vi "Target Main.vi"() -> ()   [LabVIEW 2013]
doc: "This application launches and executes the Tag Bus Data framework configuration for the specified target alias. This is a simple example of the framework API functions, but may also be a suitable starting point for a Host UI or Thick Client that is running a local version of the framework."
uses:
  <vilib>/NI/Module Execution Interface/Engine Runtime/Execution States.ctl
  <vilib>/NI/Module Execution Interface/Engine Runtime/Fault.ctl
  <vilib>/NI/Tag Bus Module Framework/runtime/error classification.ctl
  <vilib>/NI/Module Execution Interface/Engine Runtime/Engine Runtime Interface.lvclass
  <vilib>/userdefined/High Color/nirio_resource_hc.ctl
  <vilib>/NI/DCAF/Tag Editor Core/Framework Configuration Classes/target runtime/PL_Target Runtime.lvclass
  <vilib>/NI/Tag Bus Module Framework/FPGA manager/FPGA manager.lvlib
  <vilib>/rvi/interface/nirviOpenFPGA/nirviOpenFPGA.xnode
  <vilib>/NI/Tag Bus Module Framework/FPGA manager/methods.ctl
  <vilib>/NI_Real-Time Target Support.lvlib
  <vilib>/NI/Tag Bus Module Framework/runtime/TBM module execution interface.lvclass
panel:
  in  "configuration file path":path=path "/home/lvuser/DCAFshm.pcfg"
  in  "target alias":string="cRIO"
  out "engine status":T4(array[cluster])
  out "stop":bool
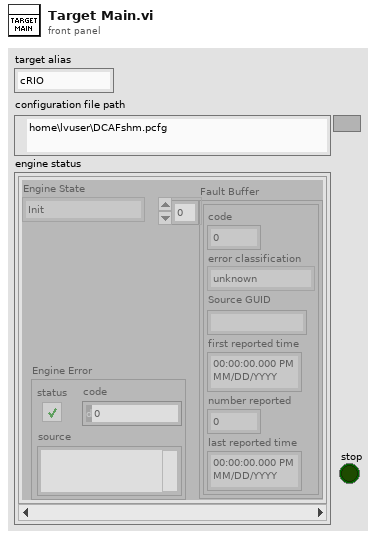
[diagram p1: front panel]
types:
  T1 = typedef "Engine Runtime Interface.lvclass/Execution States.ctl" = enum16{"Init", "Pre-Operational", "Safe-Operational", "Operational", "Stopped"}
  T2 = typedef "Engine Runtime Interface.lvclass/Fault.ctl" = cluster{"code":i32, "error classification":T3, "Source GUID":string, "first reported time":timestamp, "number reported":u32, "last reported time":timestamp}
  T3 = typedef "TBM module execution interface.lvclass/error classification.ctl" = enum16{"unknown", "none", "trivial", "recoverable", "critical"}
  T4 = cluster{"Engine State":T1, "Fault Buffer":T2[], "Engine Error":errorcluster}[]
  T5 = typedef "FPGA manager.lvlib/methods.ctl" = enum16{"initialize bitfile", "cache bitfile", "locate bitfile", "close bitfile", "clear manager"}
  T6 = typedef "nirio_resource_hc.ctl" = tag
  T7 = cluster{"Engine State":T1, "faults":T2[], "Engine Error":errorcluster}
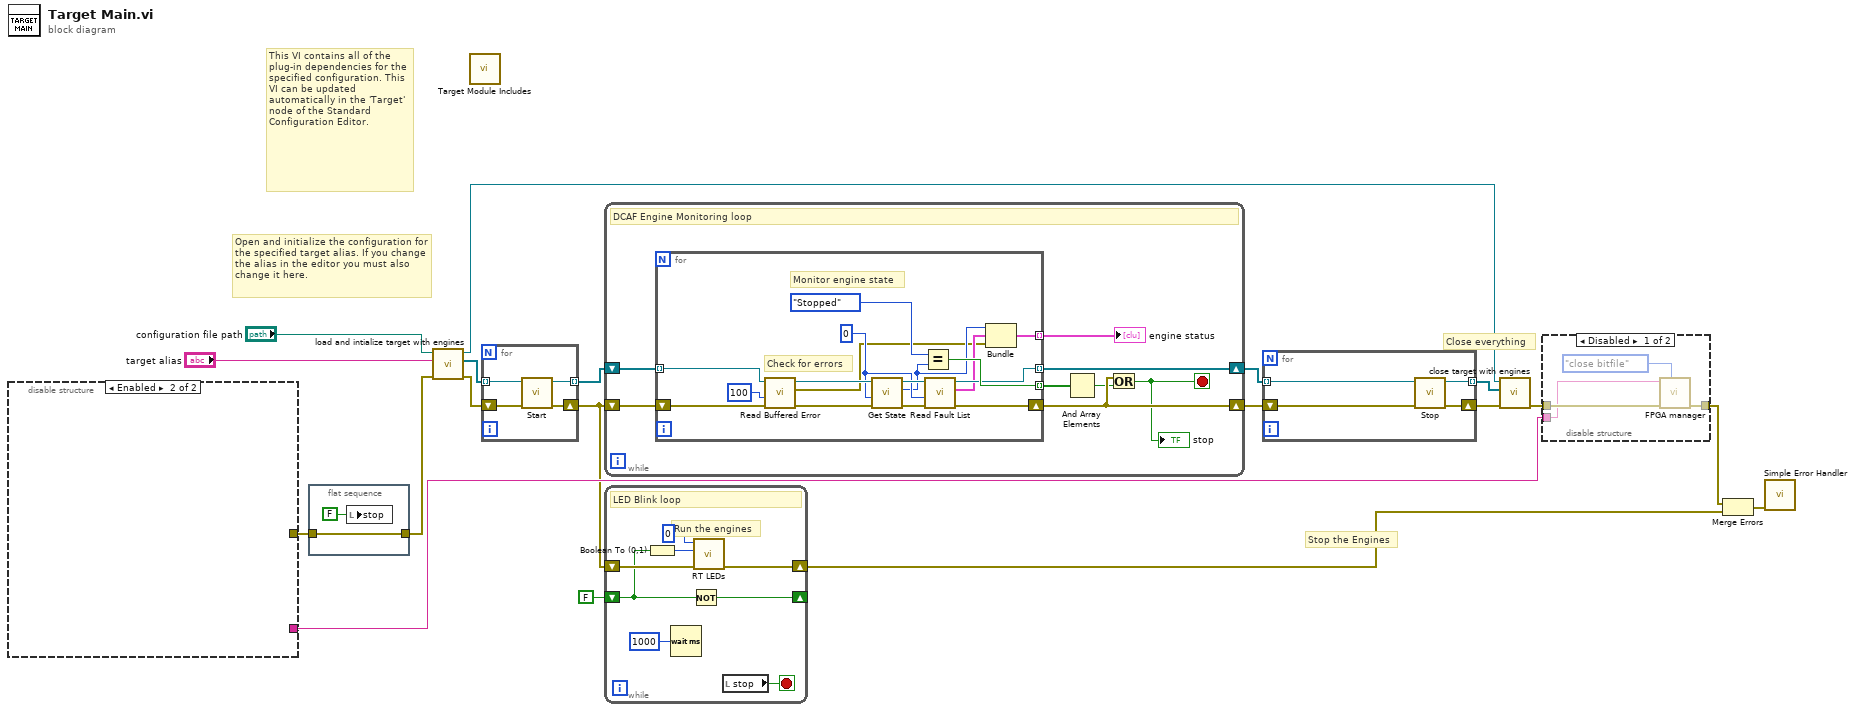
[diagram p0: block diagram]
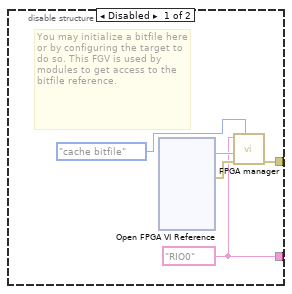
[diagram p3: hidden frame]
diagram:
  # "Open and initialize the configuration for the specified target alias. If you change the alias in the editor you must also change it here."
  # "Close everything"
  # "Stop the Engines"
  # "This VI contains all of the plug-in dependencies for the specified configuration. This VI can be updated automatically in the 'Target' node of the Standard Configuration Editor."
  # "Run the engines"
  n1 = disable-structure shown="Enabled" {
    disable-tunnel: [w24 _] -> w3
    disable-tunnel: [w20 _] -> w9
    frame Disabled {
      w20 = T6 "RIO0" ("RIO resource")
      # "You may initialize a bitfile here or by configuring the target to do so. This FGV is used by modules to get access to the bitfile reference."
      n2 = xnode "Open FPGA VI Reference"() -> ("FPGA VI Reference Out"=w22:refnum<k20>, "error out"=w23:errorcluster)  [unwired: 2 in]
      n3 = call <vilib>:"FPGA manager.vi"("action"=methods."cache bitfile", "error in"=w23, "bitfile to cache"=w22, "RIO resource"=w20) -> ("error out"=w24:errorcluster)  [unwired: 5 in, 2 out]
    }
    frame Enabled {
    }
  }
  n4 = flat-sequence {
    tunnel: w3 -> [w25]
    tunnel: [w25] -> w2
    frame #0 {
      n5 = local write "stop"(FALSE ("stop")) -> ()
    }
  }
  n6 = call <vilib>:"load and intialize target with engines.vi"("error in"=w2, "target alias"="target alias", "file path"="configuration file path") -> ("error out"=w16:errorcluster, "engine runtime interfaces"=w15:refnum<class "Engine Runtime Interface.lvclass">[], "target runtime"=w12:refnum<class "PL_Target Runtime.lvclass">)  [unwired: 6 in]
  n7 = call "Target Module Includes.vi"() -> ()  [unwired: 12 in]
  n8 = for {
    tunnel: [w30] -> w19 mode=indexing
    tunnel: w15 -> [w27] mode=indexing
    shift-right: [w29] -> w8
    shift-left: w16 -> [w28]
    n9 = call-dynamic "Start.vi"("error in"=w28, "Engine Runtime Interface in"=w27) -> ("error out"=w29:errorcluster, "Engine Runtime Interface out"=w30:refnum<class "Engine Runtime Interface.lvclass">)  [unwired: 8 in]
  }
  n10 = while {
    shift-right: [w36] -> w18
    shift-left: w19 -> [w38]
    shift-right: [w35] -> w17
    shift-left: w8 -> [w37]
    stop <- w31 stop-if-true
    # "DCAF Engine Monitoring loop"
    n11 = for {
      tunnel: w38 -> [w54] mode=indexing
      tunnel: [w45] -> w36 mode=indexing
      tunnel: [w49] -> w33 mode=indexing
      shift-right: [w44] -> w35
      shift-left: w37 -> [w53]
      tunnel: [w39] -> w34 mode=indexing
      w43 = 0 ("timeout (-1)")
      # "Monitor engine state"
      # "Check for errors"
      n12 = call-dynamic "Read Buffered Error.vi"("error in"=w53, "timeout in ms (0)"=100, "Engine Runtime Interface in"=w54) -> ("error out"=w51:errorcluster, "Engine Error"=w40:errorcluster, "Engine Runtime Interface out"=w52:refnum<class "Engine Runtime Interface.lvclass">)  [unwired: 6 in]
      n13 = call-dynamic "Get State.vi"("error in"=w51, "timeout (-1)"=w43, "Engine Runtime Interface in"=w52) -> ("error out"=w47:errorcluster, "Engine State"=w42:T1, "Engine Runtime Interface out"=w46:refnum<class "Engine Runtime Interface.lvclass">)  [unwired: 6 in]
      n14 = Equal?(x=Execution_States."Stopped" ("Engine State"), y=w42) -> (x = y?=w49:bool)
      n15 = call-dynamic "Read Fault List.vi"("error in"=w47, "timeout (-1)"=w43, "Engine Runtime Interface in"=w46) -> ("error out"=w44:errorcluster, "faults"=w41:T2[], "Engine Runtime Interface out"=w45:refnum<class "Engine Runtime Interface.lvclass">)  [unwired: 6 in]
      n16 = Bundle("Engine State"=w42, "faults"=w41, "Engine Error"=w40) -> (w39:T7)  [unwired: 1 in]
    }
    "engine status" <- w34
    n17 = And Array Elements(Boolean array=w33) -> (logical AND=w32:bool)
    n18 = Or(x=w35, y=w32) -> (x .or. y?=w31:bool)
    "stop" <- w31
  }
  n19 = while {
    shift-right: [w60] -> w7
    shift-left: w8 -> [w61]
    shift-right: [w58] -> _
    shift-left: FALSE ("stop") -> [w57]
    stop <- w55 stop-if-true
    # "LED Blink loop"
    n20 = Boolean To (0,1)(Boolean=w57) -> (0, 1=w56:i16)
    n21 = Wait (ms)(milliseconds to wait=u32 1000) -> ()  [unwired: 1 out]
    n22 = Not(x=w57) -> (.not. x?=w58:bool)
    n23 = call <vilib>:"RT LEDs.vi"("error in (no error)"=w61, "State"=w56, "LED Num"=0) -> ("error out"=w60:errorcluster)  [unwired: 3 in, 1 out]
    n24 = local read "stop"() -> (w55:bool)
  }
  n25 = for {
    tunnel: w18 -> [w66] mode=indexing
    shift-right: [w63] -> w11
    shift-left: w17 -> [w65]
    tunnel: [w64] -> w13 mode=indexing
    n26 = call-dynamic "Stop.vi"("error in"=w65, "Engine Runtime Interface in"=w66) -> ("error out"=w63:errorcluster, "Engine Runtime Interface out"=w64:refnum<class "Engine Runtime Interface.lvclass">)  [unwired: 8 in]
  }
  n27 = call <vilib>:"close target with engines.vi"("error in"=w11, "Engine Runtime Interfaces"=w13, "Target Runtime"=w12) -> ("error out"=w6:errorcluster)  [unwired: 8 in]
  n28 = disable-structure shown="Disabled" {
    disable-tunnel: [w69 w71] -> w5
    disable-tunnel: w6 -> [w70 w71]
    disable-tunnel: w9 -> [w67 _]
    frame Disabled {
      n29 = call <vilib>:"FPGA manager.vi"("action"=methods."close bitfile", "error in"=w70, "RIO resource"=w67) -> ("error out"=w69:errorcluster)  [unwired: 6 in, 2 out]
    }
    frame Enabled {
    }
  }
  n30 = Merge Errors(w5, w7) -> (w4:errorcluster)
  n31 = call <vilib>:"Simple Error Handler.vi"("error in (no error)"=w4) -> ()  [unwired: 4 in, 5 out]
